vi "DAQmx-AI.SetLogging.vi"(8 "error in (no error)":errorcluster, 9 "Group Name":string, 10 "TDMS File Path":path, 11 "DAQmx-AI":refnum<class "DAQmx-AI.lvclass">) -> (0 "error out":errorcluster, 3 "DAQmx-AI out":refnum<class "DAQmx-AI.lvclass">)   [LabVIEW 2016, in "DAQmx-AI.lvclass"]
uses:
  DAQmx-AI.lvclass
  DAQmx-AI.lvclass/DAQmx-AI.ctl
  Typedefs/Logging--Cluster.ctl
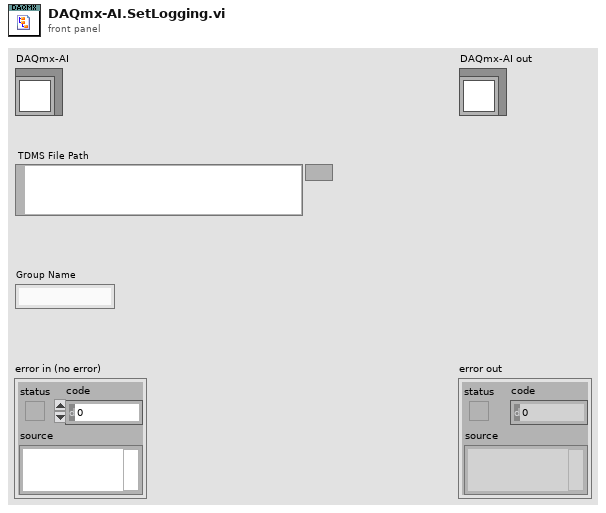
[diagram p1: front panel]
types:
  T1 = typedef "DAQmx-AI.lvclass/Logging--Cluster.ctl" = cluster{"TDMS File Path":path, "Group Name":string}
  T2 = typedef "DAQmx-AI.lvclass/PrivateData--Ref.ctl" = refnum<data-value>
  T3 = typedef "DAQmx-AI.lvclass/PrivateData--Cluster.ctl" = cluster{"Configuration":T4, "Public Events":T6, "Data":dbl, "Scaling":T7, "Private Events":T13}
  T4 = typedef "DAQmx-AI.lvclass/Configuration--Cluster.ctl" = cluster{"PhysChan":tag, "Period (ms)":i64, "input terminal cfg":i32, "minimum value":dbl, "maximum value":dbl, "units":T5, "task name":string, "TDMS File Path":path, "Group Name":string}
  T5 = typedef "DAQmx-AI.lvclass/Units -- Enum.ctl" = enum16{"Volts", "Amps", "Deg F", "Deg C", "Deg R", "Kelvins", "Strain", "Ohms", "Hz", "Seconds", "Meters", "Inches", "Degrees", "Radians", "Ticks", "g", "m/s^2", "m/s", "in/s", "Pascals", "Newtons", "Pounds", "kgf", "psi", "bar", "Nm", "oz-in", "lb-in", "lb-ft", "Volts/Volt", "mVolts/Volt", "From TEDS"}
  T6 = typedef "DAQmx-AI.lvclass/PublicEvents--Cluster.ctl" = cluster{"Value Changed":refnum<user-event>, "Task Configuration":refnum<user-event>, "Scaling":refnum<user-event>}
  T7 = typedef "DAQmx-AI.lvclass/Scaling--Cluster.ctl" = cluster{"Scale Name":string, "Scale Type":T8, "Scaled Units":string, "Linear":T9, "Map Range":T10, "Polynomial":T11, "Table":T12}
  T8 = typedef "DAQmx-AI.lvclass/ScalingType--Enum.ctl" = enum16{"No scaling", "Linear", "Map Range", "Polynomial", "Table"}
  T9 = typedef "DAQmx-AI.lvclass/Scaling(Linear)--Cluster.ctl" = cluster{"Slope":dbl, "Intercept":dbl}
  T10 = typedef "DAQmx-AI.lvclass/Scaling(MapRange)--Cluster.ctl" = cluster{"Minimum":dbl, "Maximum":dbl}
  T11 = typedef "DAQmx-AI.lvclass/Scaling(Polynomial)--Cluster.ctl" = cluster{"forward coeff":dbl[], "reverse coeff":dbl[]}
  T12 = typedef "DAQmx-AI.lvclass/Scaling(Table)--Cluster.ctl" = cluster{"scaled values":dbl[], "pres-scaled values":dbl[]}
  T13 = typedef "DAQmx-AI.lvclass/PrivateEvents--Cluster.ctl" = cluster{"Logging":refnum<user-event>}
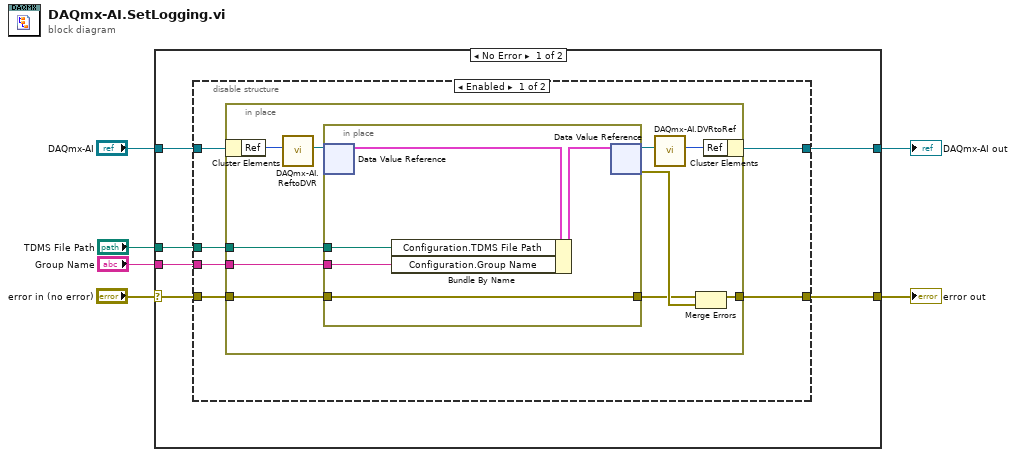
[diagram p0: block diagram]
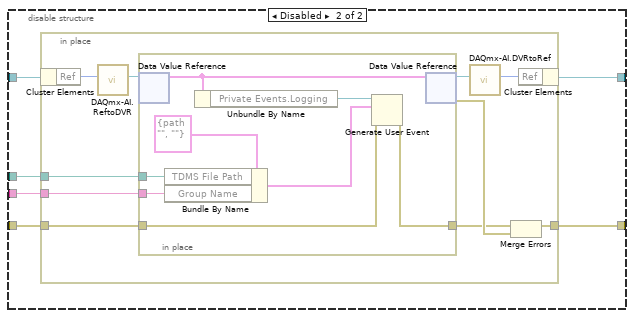
[diagram p2: hidden frame]
diagram:
  n1 = case shown="No Error" "error in (no error)" {
    selector: "error in (no error)" -> [w8 w59]
    tunnel: [w7 w59] -> w5
    tunnel: [w10 w58] -> w3
    tunnel: "DAQmx-AI" -> [w11 w58]
    tunnel: "TDMS File Path" -> [w12 _]
    tunnel: "Group Name" -> [w9 _]
    frame No Error {
      n2 = disable-structure shown="Enabled" {
        disable-tunnel: w12 -> [w14 w35]
        disable-tunnel: [w17 w38] -> w10
        disable-tunnel: w11 -> [w18 w39]
        disable-tunnel: w9 -> [w13 w34]
        disable-tunnel: w8 -> [w16 w37]
        disable-tunnel: [w15 w36] -> w7
        frame Enabled {
          n3 = in-place {
            in-place-border: w16 -> [w28]
            in-place-border: [w25] -> w15
            in-place-border: w14 -> [w20]
            in-place-border: w13 -> [w19]
            n4 = in-place-cluster #1(w18) -> ("Ref"=w24:u32)
            n5 = call "DAQmx-AI.ReftoDVR.vi"("Ref"=w24) -> ("Ref"=w23:T2)  [unwired: 10 in]
            n6 = in-place {
              in-place-border: w28 -> [w31]
              in-place-border: [w31] -> w26
              in-place-border: w20 -> [w33]
              in-place-border: w19 -> [w32]
              n7 = in-place-dvr #2(w23) -> (w30:T3)  [unwired: 1 out]
              n8 = Bundle By Name(cluster=w30, "Configuration.TDMS File Path"=w33, "Configuration.Group Name"=w32) -> (w29:T3)
              n9 = in-place-dvr #2(w29) -> (w22:T2, w27:errorcluster)
            }
            n10 = call "DAQmx-AI.DVRtoRef.vi"("Ref"=w22) -> ("Ref"=w21:u32)  [unwired: 10 in]
            n11 = Merge Errors(w26, w27) -> (w25:errorcluster)
            n12 = in-place-cluster #1("Ref"=w21) -> (w17:refnum<class "DAQmx-AI.lvclass">)
          }
        }
        frame Disabled {
          n13 = in-place {
            in-place-border: w37 -> [w49]
            in-place-border: [w46] -> w36
            in-place-border: w35 -> [w41]
            in-place-border: w34 -> [w40]
            n14 = in-place-cluster #3(w39) -> ("Ref"=w45:u32)
            n15 = call "DAQmx-AI.ReftoDVR.vi"("Ref"=w45) -> ("Ref"=w44:T2)  [unwired: 10 in]
            n16 = in-place {
              in-place-border: w49 -> [w51]
              in-place-border: [w50] -> w47
              in-place-border: w41 -> [w55]
              in-place-border: w40 -> [w54]
              n17 = in-place-dvr #4(w44) -> (w57:T3)  [unwired: 1 out]
              n18 = Bundle By Name(cluster=T1 {"TDMS File Path"=path "", "Group Name"=""} ("Logging"), "TDMS File Path"=w55, "Group Name"=w54) -> (w52:T1)
              n19 = Unbundle By Name(w57) -> ("Private Events.Logging"=w53:refnum<user-event>)
              n20 = Generate User Event(user event=w53, event data cluster=w52, error in=w51) -> (error out=w50:errorcluster)  [unwired: 1 in, 1 out]
              n21 = in-place-dvr #4(w57) -> (w43:T2, w48:errorcluster)
            }
            n22 = call "DAQmx-AI.DVRtoRef.vi"("Ref"=w43) -> ("Ref"=w42:u32)  [unwired: 10 in]
            n23 = Merge Errors(w47, w48) -> (w46:errorcluster)
            n24 = in-place-cluster #3("Ref"=w42) -> (w38:refnum<class "DAQmx-AI.lvclass">)
          }
        }
      }
    }
    frame Error {
    }
  }
  "error out" <- w5
  "DAQmx-AI out" <- w3
